vi "FTW-Connector-Ping.vi"(0 "FTW Actor Connector":refnum<class "FTW-ActorConnector.lvclass">, 7 "Request Body":string, 9 "Timeout":i32=100 format="%dmsec", 11 "error in":errorcluster) -> (4 "FTW Actor Connector out":refnum<class "FTW-ActorConnector.lvclass">, 8 "Response Body":string, 10 "Timed out?":bool, 14 "Roundtrip Time":dbl format="%.6fsec", 15 "error out":errorcluster)   [LabVIEW 2013, in "FTW-ActorConnector.lvclass"]
uses:
  FTW-ActorConnector.lvclass
  FTW-ActorConnector.lvclass/FTW-ActorConnector.ctl
  Request/FTW-Request.lvclass
panel:
  # "Inputs"
  # "Outputs"
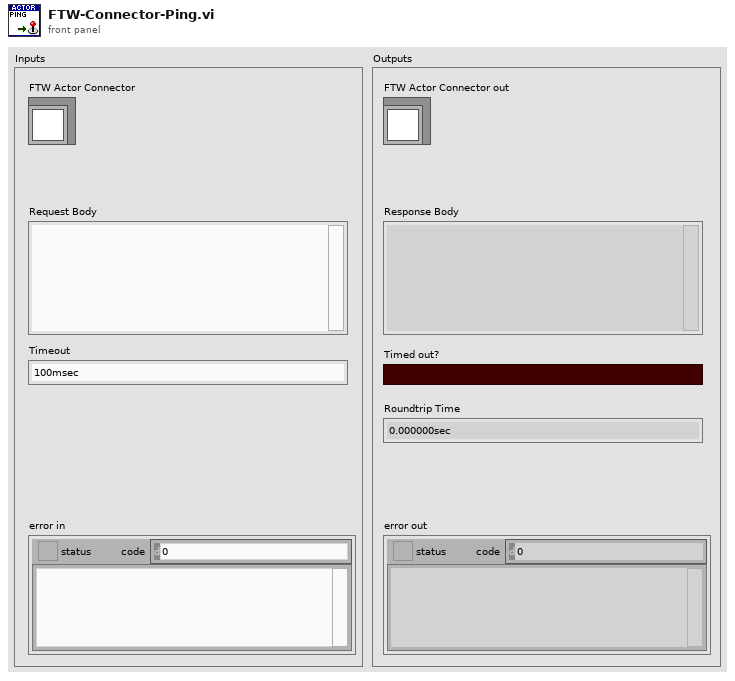
[diagram p1: front panel]
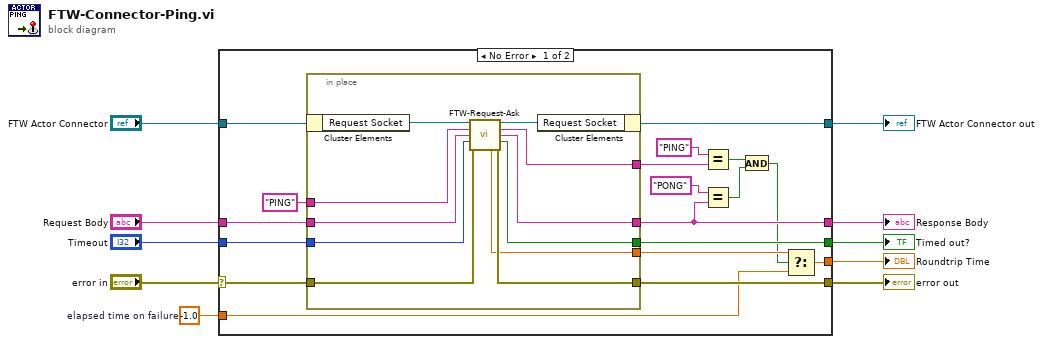
[diagram p0: block diagram]
diagram:
  w1 = -1.0  # elapsed time on failure
  n1 = case shown="No Error" "error in" {
    selector: "error in" -> [w27 w42]
    tunnel: [w25 w42] -> w9
    tunnel: "FTW Actor Connector" -> [w28 w41]
    tunnel: [w26 w41] -> w7
    tunnel: "Request Body" -> [w24 _]
    tunnel: [w23 _] -> w6
    tunnel: "Timeout" -> [w22 _]
    tunnel: [w15 _] -> w3
    tunnel: [w20 w40] -> w2
    tunnel: w1 -> [w19 w40]
    frame No Error {
      n2 = in-place {
        in-place-border: w27 -> [w39]
        in-place-border: [w38] -> w25
        in-place-border: "PING" ("Request Header") -> [w35]
        in-place-border: w24 -> [w34]
        in-place-border: [w36] -> w23
        in-place-border: w22 -> [w33]
        in-place-border: [w32] -> w15
        in-place-border: [w30] -> w16
        in-place-border: [w29] -> w13
        n3 = in-place-cluster #1(w28) -> ("Request Socket"=w31:refnum<class "FTW-Request.lvclass">)
        n4 = call "FTW-Request-Ask.vi"("FTW-Request In"=w31, "Header"=w35, "Body"=w34, "Timeout"=w33, "error in"=w39) -> ("FTW-Request Out"=w37:refnum<class "FTW-Request.lvclass">, "Response Header"=w29:string, "Response Body"=w32:string, "Timed out?"=w36:bool, "Roundtrip Time"=w30:dbl, "error out"=w38:errorcluster)  [unwired: 5 in]
        n5 = in-place-cluster #1("Request Socket"=w37) -> (w26:refnum<class "FTW-ActorConnector.lvclass">)
      }
      n6 = Equal?(x="PING", y=w13) -> (x = y?=w11:bool)
      n7 = Equal?(x="PONG", y=w15) -> (x = y?=w17:bool)
      n8 = And(x=w11, y=w17) -> (x .and. y?=w12:bool)
      n9 = Select(t=w16, s=w12, f=w19) -> (s? t:f=w20:dbl)
    }
    frame Error {
    }
  }
  "error out" <- w9
  "FTW Actor Connector out" <- w7
  "Timed out?" <- w6
  "Response Body" <- w3
  "Roundtrip Time" <- w2
